vi "Write State.vi"(8 "error in (no error)":errorcluster, 10 "State":T1, 11 "UniStableShutter in":refnum<class "UniStableShutter.lvclass">) -> (0 "error out":errorcluster, 3 "UniStableShutter out":refnum<class "UniStableShutter.lvclass">)   [LabVIEW 2016, in "UniStableShutter.lvclass"]
uses:
  UniStableShutter.lvclass
  Controls/Shutter States.ctl
  Shutter.lvclass
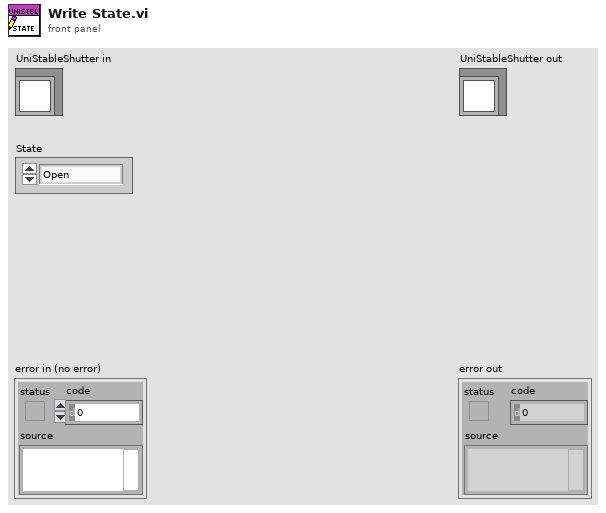
[diagram p1: front panel]
types:
  T1 = typedef "Shutter States.ctl" = enum16{"Open", "Close", "Wait", "Off", "Arm", "Idle"}
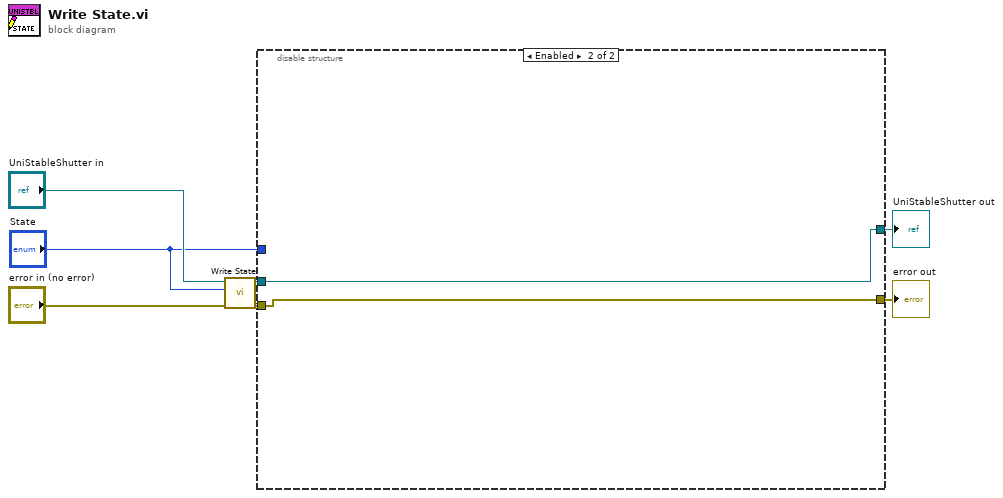
[diagram p0: block diagram]
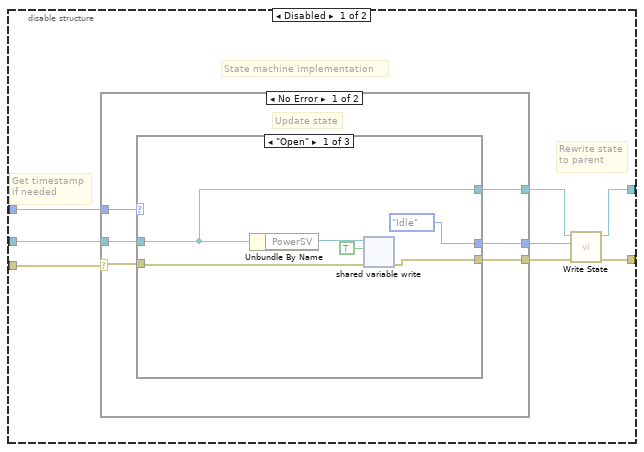
[diagram p2: hidden frame]
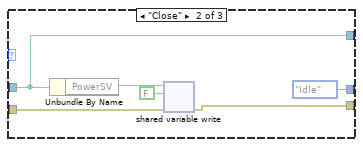
[diagram p3: hidden frame]
diagram:
  n1 = call-parent "Write State.vi"("error in (no error)"="error in (no error)", "Set"="State", "Shutter in"="UniStableShutter in") -> ("error out"=w3:errorcluster, "Shutter out"=w5:refnum<class "UniStableShutter.lvclass">)  [unwired: 7 in]
  n2 = disable-structure shown="Enabled" {
    disable-tunnel: w5 -> [w15 w41]
    disable-tunnel: "State" -> [w14 _]
    disable-tunnel: w3 -> [w13 w40]
    disable-tunnel: [w11 w40] -> w2
    disable-tunnel: [w9 w41] -> w1
    frame Disabled {
      # "Rewrite state\nto parent"
      # "Get timestamp\nif needed"
      # "State machine implementation"
      n3 = case shown="No Error" w13 {
        selector: w13 -> [w18 w39]
        tunnel: w15 -> [w21 w38]
        tunnel: w14 -> [w20 w37]
        tunnel: [w19 w38] -> w10
        tunnel: [w17 w39] -> w12
        tunnel: [w16 w37] -> w8
        frame No Error {
          # "Update state"
          n4 = case shown="\"Open\"" w20 {
            selector: w20 -> [_ _ w34]
            tunnel: w21 -> [w23 w29 w36]
            tunnel: [w23 w29 w36] -> w19
            tunnel: w18 -> [w25 w31 w35]
            tunnel: [w24 w30 w35] -> w17
            tunnel: [Shutter_States."Idle" ("Set") Shutter_States."Idle" ("Set") w34] -> w16
            frame "Open" {
              n5 = Unbundle By Name(w23) -> ("PowerSV"=w27:refnum<k21>)
              n6 = shared-variable-write(w27, w25, TRUE ("data in")) -> (w24:errorcluster)  [unwired: 1 out]
            }
            frame "Close" {
              n7 = Unbundle By Name(w29) -> ("PowerSV"=w33:refnum<k21>)
              n8 = shared-variable-write(w33, w31, FALSE ("data in")) -> (w30:errorcluster)  [unwired: 1 out]
            }
            frame Default {
            }
          }
        }
        frame Error {
        }
      }
      n9 = call-parent "Write State.vi"("error in (no error)"=w12, "Set"=w8, "Shutter in"=w10) -> ("error out"=w11:errorcluster, "Shutter out"=w9:refnum<class "UniStableShutter.lvclass">)  [unwired: 7 in]
    }
    frame Enabled {
    }
  }
  "error out" <- w2
  "UniStableShutter out" <- w1
